vi "Tote Autonomous.vi"   [LabVIEW 2014]
uses:
  <vilib>/Rock Robotics/WPI/RobotDrive/WPI_RobotDriveGetSetRefNum.vi
types:
  T1 = typedef "WPI_MotorControlDeviceRef.ctl" = cluster{"DeviceStatus":errorcluster, "Type":T2, "PWM":cluster{"Controller":T3, "PWM Channel":T4, "DeadBand":T5}, "CAN":cluster{"Device Number":u8, "Control Mode":T6, "Semaphore":T7, "Max Vout":dbl, "TalonSRX Control Mode":T8}, "Invert":bool, "TransformRef":T9, "InvTransformRef":T9}
  T2 = typedef "WPI_MotorControlType.ctl" = enum16{"PWM", "CAN", "CANTalonSRX"}
  T3 = typedef "FPGA_TypedefDigitalModule.ctl" = enum16{"Controller 1"}
  T4 = typedef "FPGA_DIOPWMChannel.ctl" = enum8{"PWM 0", "PWM 1", "PWM 2", "PWM 3", "PWM 4", "PWM 5", "PWM 6", "PWM 7", "PWM 8", "PWM 9", "PWM MXP 0", "PWM MXP 1", "PWM MXP 2", "PWM MXP 3", "PWM MXP 4", "PWM MXP 5", "PWM MXP 6", "PWM MXP 7", "PWM MXP 8", "PWM MXP 9", "Invalid"}
  T5 = typedef "WPI_PWMDeadband.ctl" = cluster{"Name":string, "maxPositivePwm":i32, "minPositivePwm":i32, "centerPwm":i32, "maxNegativePwm":i32, "minNegativePwm":i32, "angularRange":u16}
  T6 = typedef "WPI_CANJaguar_ControlMode.ctl" = enum8{"Percent VBus", "Current", "Speed", "Position", "Voltage"}
  T7 = typedef "Semaphore RefNum" = refnum<k1>
  T8 = typedef "WPI_CANTalonSRX_APIControlMode.ctl" = enum8{"Percent VBus", "Speed", "Position", "Slave", "Unchanged / Invalid"}
  T9 = typedef "WPI_PWMTransform_ConPane.ctl" = refnum<vi>
  T10 = typedef "WPI_EncoderDevRef.ctl" = cluster{"DevStatus":errorcluster, "EncoderIndex":T11, "CounterIndex":T12, "DistancePerCount":dbl, "Decoding Type":T13}
  T11 = typedef "FPGA_EncoderIdx.ctl" = enum8{"Enc 0", "Enc 1", "Enc 2", "Enc 3", "Enc 4", "Enc 5", "Enc 6", "Enc 7", "Invalid"}
  T12 = typedef "FPGA_CounterCtrSystemIndex.ctl" = enum8{"Ctr 0", "Ctr 1", "Ctr 2", "Ctr 3", "Ctr 4", "Ctr 5", "Ctr 6", "Ctr 7", "Invalid"}
  T13 = typedef "WPI_EncoderType.ctl" = enum16{"1x", "2x", "4x"}
  T14 = typedef "WPI_RobotDriveDevRef.ctl" = cluster{"DevStatus":errorcluster, "Motors[]":T1[], "Square Inputs":bool, "Max Output":dbl}
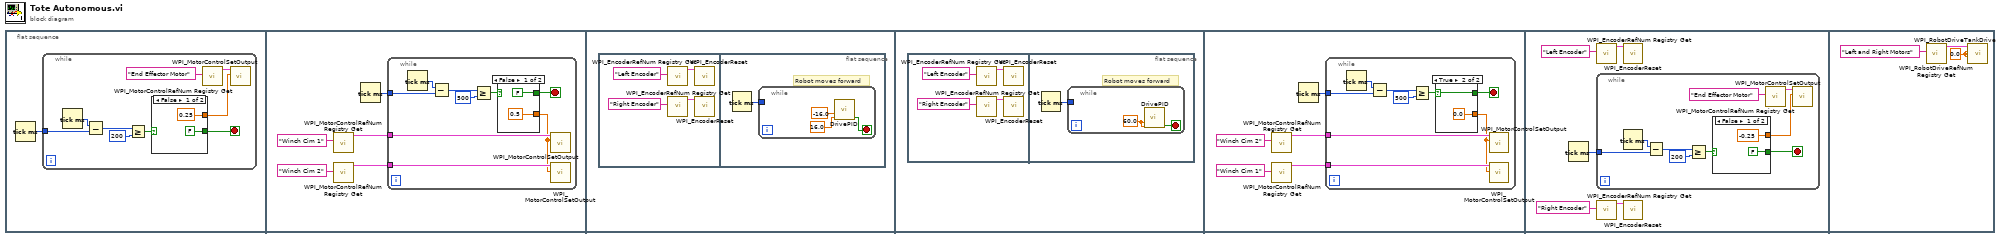
[diagram p0: block diagram]
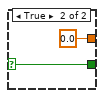
[diagram p2: hidden frame]
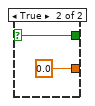
[diagram p3: hidden frame]
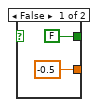
[diagram p4: hidden frame]
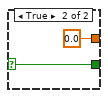
[diagram p5: hidden frame]
diagram:
  n1 = flat-sequence {
    frame #0 {
      n2 = Tick Count (ms)() -> (millisecond timer value=w1:u32)
      n3 = while {
        tunnel: w1 -> [w8]
        stop <- w3 stop-if-true
        n4 = Tick Count (ms)() -> (millisecond timer value=w9:u32)
        n5 = Subtract(x=w9, y=w8) -> (x-y=w7:u32)
        n6 = Greater Or Equal?(x=w7, y=u32 200) -> (x >= y?=w6:bool)
        n7 = case shown="False" w6 {
          selector: w6 -> [_ w13]
          tunnel: [0.25 ("Output") 0.0 ("Output")] -> w4
          tunnel: [FALSE w13] -> w3
          frame False {
          }
          frame True {
          }
        }
        n8 = call <vilib>:"WPI_MotorControlRefNum Registry Get.vi"("refnum name"="End Effector Motor") -> ("MotorControlDevRef"=w5:T1)  [unwired: 9 in, 1 out]
        n9 = call <vilib>:"WPI_MotorControlSetOutput.vi"("Output"=w4, "MotorControlDevRef"=w5) -> ()  [unwired: 7 in, 3 out]
      }
    }
    frame #1 {
      n10 = call <vilib>:"WPI_MotorControlRefNum Registry Get.vi"("refnum name"="Winch Cim 1") -> ("MotorControlDevRef"=w19:T1)  [unwired: 9 in, 1 out]
      n11 = call <vilib>:"WPI_MotorControlRefNum Registry Get.vi"("refnum name"="Winch Cim 2") -> ("MotorControlDevRef"=w16:T1)  [unwired: 9 in, 1 out]
      n12 = Tick Count (ms)() -> (millisecond timer value=w15:u32)
      n13 = while {
        tunnel: w19 -> [w24]
        tunnel: w16 -> [w23]
        tunnel: w15 -> [w25]
        stop <- w20 stop-if-true
        n14 = Tick Count (ms)() -> (millisecond timer value=w26:u32)
        n15 = Subtract(x=w26, y=w25) -> (x-y=w28:u32)
        n16 = Greater Or Equal?(x=w28, y=u32 500) -> (x >= y?=w22:bool)
        n17 = case shown="False" w22 {
          selector: w22 -> [_ w31]
          tunnel: [0.5 ("Output") 0.0 ("Output")] -> w21
          tunnel: [FALSE w31] -> w20
          frame False {
          }
          frame True {
          }
        }
        n18 = call <vilib>:"WPI_MotorControlSetOutput.vi"("Output"=w21, "MotorControlDevRef"=w24) -> ()  [unwired: 7 in, 3 out]
        n19 = call <vilib>:"WPI_MotorControlSetOutput.vi"("Output"=w21, "MotorControlDevRef"=w23) -> ()  [unwired: 7 in, 3 out]
      }
    }
    frame #2 {
      n20 = flat-sequence {
        frame #0 {
          n21 = call <vilib>:"WPI_EncoderRefNum Registry Get.vi"("refnum name"="Left Encoder") -> ("EncoderDevRef"=w34:T10)  [unwired: 9 in, 1 out]
          n22 = call <vilib>:"WPI_EncoderRefNum Registry Get.vi"("refnum name"="Right Encoder") -> ("EncoderDevRef"=w36:T10)  [unwired: 9 in, 1 out]
          n23 = call <vilib>:"WPI_EncoderReset.vi"("EncoderDevRef"=w34) -> ()  [unwired: 9 in, 2 out]
          n24 = call <vilib>:"WPI_EncoderReset.vi"("EncoderDevRef"=w36) -> ()  [unwired: 9 in, 2 out]
        }
        frame #1 {
          # "Robot moves forward"
          n25 = Tick Count (ms)() -> (millisecond timer value=w37:u32)
          n26 = while {
            tunnel: w37 -> [_]
            stop <- w40 stop-if-true
            n27 = call "DrivePID.vi"("SetpointRight"=-16.0, "SetpointLeft"=16.0) -> ("Done"=w40:bool)  [unwired: 13 in]
          }
        }
      }
    }
    frame #3 {
      n28 = flat-sequence {
        frame #0 {
          n29 = call <vilib>:"WPI_EncoderRefNum Registry Get.vi"("refnum name"="Left Encoder") -> ("EncoderDevRef"=w42:T10)  [unwired: 9 in, 1 out]
          n30 = call <vilib>:"WPI_EncoderRefNum Registry Get.vi"("refnum name"="Right Encoder") -> ("EncoderDevRef"=w44:T10)  [unwired: 9 in, 1 out]
          n31 = call <vilib>:"WPI_EncoderReset.vi"("EncoderDevRef"=w42) -> ()  [unwired: 9 in, 2 out]
          n32 = call <vilib>:"WPI_EncoderReset.vi"("EncoderDevRef"=w44) -> ()  [unwired: 9 in, 2 out]
        }
        frame #1 {
          # "Robot moves forward"
          n33 = Tick Count (ms)() -> (millisecond timer value=w45:u32)
          n34 = while {
            tunnel: w45 -> [_]
            stop <- w46 stop-if-true
            w47 = 60.0 ("SetpointRight")
            n35 = call "DrivePID.vi"("SetpointRight"=w47, "SetpointLeft"=w47) -> ("Done"=w46:bool)  [unwired: 13 in]
          }
        }
      }
    }
    frame #4 {
      n36 = call <vilib>:"WPI_MotorControlRefNum Registry Get.vi"("refnum name"="Winch Cim 2") -> ("MotorControlDevRef"=w49:T1)  [unwired: 9 in, 1 out]
      n37 = call <vilib>:"WPI_MotorControlRefNum Registry Get.vi"("refnum name"="Winch Cim 1") -> ("MotorControlDevRef"=w52:T1)  [unwired: 9 in, 1 out]
      n38 = Tick Count (ms)() -> (millisecond timer value=w48:u32)
      n39 = while {
        tunnel: w52 -> [w57]
        tunnel: w49 -> [w56]
        tunnel: w48 -> [w58]
        stop <- w53 stop-if-true
        n40 = Tick Count (ms)() -> (millisecond timer value=w59:u32)
        n41 = Subtract(x=w59, y=w58) -> (x-y=w61:u32)
        n42 = Greater Or Equal?(x=w61, y=u32 500) -> (x >= y?=w55:bool)
        n43 = case shown="True" w55 {
          selector: w55 -> [_ w64]
          tunnel: [-0.5 ("Output") 0.0 ("Output")] -> w54
          tunnel: [FALSE w64] -> w53
          frame False {
          }
          frame True {
          }
        }
        n44 = call <vilib>:"WPI_MotorControlSetOutput.vi"("Output"=w54, "MotorControlDevRef"=w56) -> ()  [unwired: 7 in, 3 out]
        n45 = call <vilib>:"WPI_MotorControlSetOutput.vi"("Output"=w54, "MotorControlDevRef"=w57) -> ()  [unwired: 7 in, 3 out]
      }
    }
    frame #5 {
      n46 = Tick Count (ms)() -> (millisecond timer value=w66:u32)
      n47 = call <vilib>:"WPI_EncoderRefNum Registry Get.vi"("refnum name"="Left Encoder") -> ("EncoderDevRef"=w68:T10)  [unwired: 9 in, 1 out]
      n48 = while {
        tunnel: w66 -> [w77]
        stop <- w71 stop-if-true
        n49 = Tick Count (ms)() -> (millisecond timer value=w78:u32)
        n50 = Subtract(x=w78, y=w77) -> (x-y=w76:u32)
        n51 = Greater Or Equal?(x=w76, y=u32 200) -> (x >= y?=w74:bool)
        n52 = case shown="False" w74 {
          selector: w74 -> [_ w82]
          tunnel: [-0.25 ("Output") 0.0 ("Output")] -> w72
          tunnel: [FALSE w82] -> w71
          frame False {
          }
          frame True {
          }
        }
        n53 = call <vilib>:"WPI_MotorControlRefNum Registry Get.vi"("refnum name"="End Effector Motor") -> ("MotorControlDevRef"=w73:T1)  [unwired: 9 in, 1 out]
        n54 = call <vilib>:"WPI_MotorControlSetOutput.vi"("Output"=w72, "MotorControlDevRef"=w73) -> ()  [unwired: 7 in, 3 out]
      }
      n55 = call <vilib>:"WPI_EncoderRefNum Registry Get.vi"("refnum name"="Right Encoder") -> ("EncoderDevRef"=w70:T10)  [unwired: 9 in, 1 out]
      n56 = call <vilib>:"WPI_EncoderReset.vi"("EncoderDevRef"=w68) -> ()  [unwired: 9 in, 2 out]
      n57 = call <vilib>:"WPI_EncoderReset.vi"("EncoderDevRef"=w70) -> ()  [unwired: 9 in, 2 out]
    }
    frame #6 {
      w84 = 0.0 ("Left axis value")
      n58 = call <vilib>:"WPI_RobotDriveRefNum Registry Get.vi"("refnum name"="Left and Right Motors") -> ("RobotDriveDevRef"=w85:T14)  [unwired: 9 in, 1 out]
      n59 = call <vilib>:"WPI_RobotDriveTankDrive.vi"("Right axis value"=w84, "Left axis value"=w84, "RobotDriveDevRef"=w85) -> ()  [unwired: 6 in, 3 out]
    }
  }
